vi "Read Timeout Event State Ref.vi"(8 "error in (no error)":errorcluster, 11 "CSM-Helper in":refnum<class "CSM-Helper.lvclass">) -> (0 "error out":errorcluster, 1 "New State Notifier Event State Ref":refnum<vi>, 3 "CSM-Helper out":refnum<class "CSM-Helper.lvclass">)   [LabVIEW 2017, in "CSM-Helper.lvclass"]
doc: "### Read Timeout Event State Ref.vi\n\n-- <b>Controls</b> --\n- <b>CSM-Helper in</b>: CSMHelper input\n\n-- <b>Indicators</b> --\n- <b>New State Notifier Event State Ref</b>:\n- <b>CSM-Helper out</b>: CSMHelper output"
uses:
  CSM-Helper.lvclass
  CSM-Helper.lvclass/CSM-Helper.ctl
  _Shared/CSM Shared.lvlib
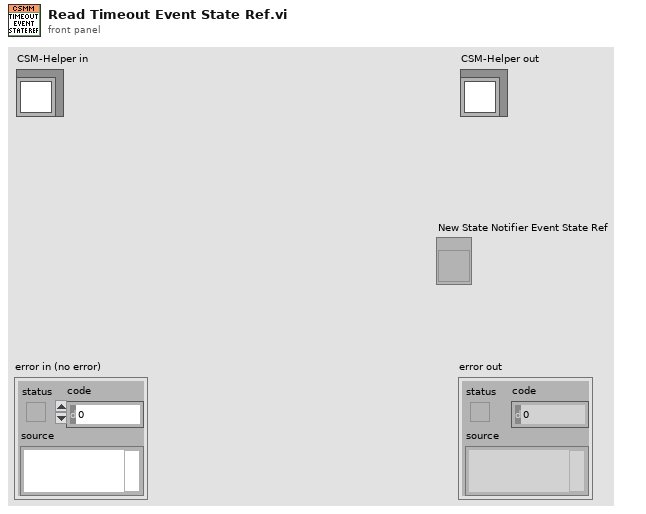
[diagram p1: front panel]
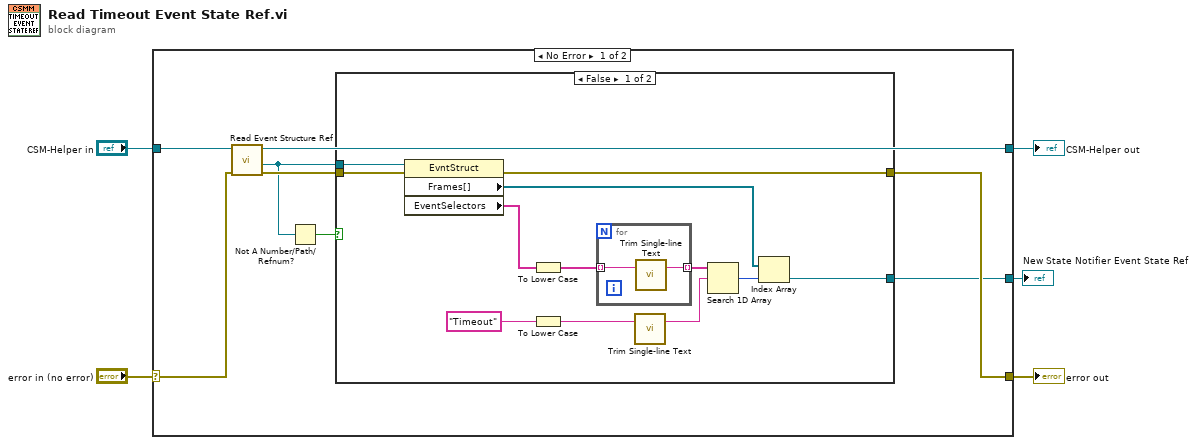
[diagram p0: block diagram]
diagram:
  n1 = case shown="No Error" "error in (no error)" {
    selector: "error in (no error)" -> [w11 w30]
    tunnel: [w9 w30] -> w4
    tunnel: [w12 w29] -> w2
    tunnel: "CSM-Helper in" -> [w13 w29]
    tunnel: [w6 _] -> w1
    frame No Error {
      n2 = call "Read Event Structure Ref.vi"("error in (no error)"=w11, "CSM-Helper in"=w13) -> ("error out"=w10:errorcluster, "Event Structure"=w8:refnum<vi>, "CSM-Helper out"=w12:refnum<class "CSM-Helper.lvclass">)  [unwired: 7 in]
      n3 = Not A Number/Path/Refnum?(number/path/refnum=w8) -> (NaN/Path/Refnum?=w7:bool)
      n4 = case shown="False" w7 {
        tunnel: w10 -> [w25 w28]
        tunnel: [w24 w28] -> w9
        tunnel: w8 -> [w23 _]
        tunnel: [w14 _] -> w6
        frame False {
          n5 = property class="EvntStruct"(reference=w23, error in=w25) -> (error out=w24:errorcluster, "Frames[]"=w15:refnum<vi>[], "EventSelectors"=w22:string[])  [unwired: 1 out]
          n6 = To Lower Case(string=w22) -> (all lower case string=w20:string[])
          n7 = To Lower Case(string="Timeout" ("element")) -> (all lower case string=w19:string)
          n8 = for {
            tunnel: w20 -> [w27] mode=indexing
            tunnel: [w26] -> w17 mode=indexing
            n9 = call "Trim Single-line Text.vi"("single-line text"=w27) -> ("trimed text"=w26:string)  [unwired: 2 in]
          }
          n10 = call "Trim Single-line Text.vi"("single-line text"=w19) -> ("trimed text"=w18:string)  [unwired: 2 in]
          n11 = Search 1D Array(1D array=w17, element=w18) -> (index of element=w16:i32)  [unwired: 1 in]
          n12 = Index Array(array=w15, index=w16) -> (element=w14:refnum<vi>)
        }
        frame True {
        }
      }
    }
    frame Error {
    }
  }
  "error out" <- w4
  "CSM-Helper out" <- w2
  "New State Notifier Event State Ref" <- w1
